vi "Read byte orders.vi"(8 "error in":errorcluster, 11 "Profibus Module configuration in":refnum<class "Profibus Module configuration.lvclass">) -> (0 "error out":errorcluster, 2 "byte orders":T1[](array[typedef]), 3 "Profibus Module configuration out":refnum<class "Profibus Module configuration.lvclass">)   [LabVIEW 2013, in "Profibus Module configuration.lvclass"]
uses:
  Profibus Module configuration.lvclass
  endianness setting.ctl
  Profibus Module configuration.lvclass/Profibus Module configuration.ctl
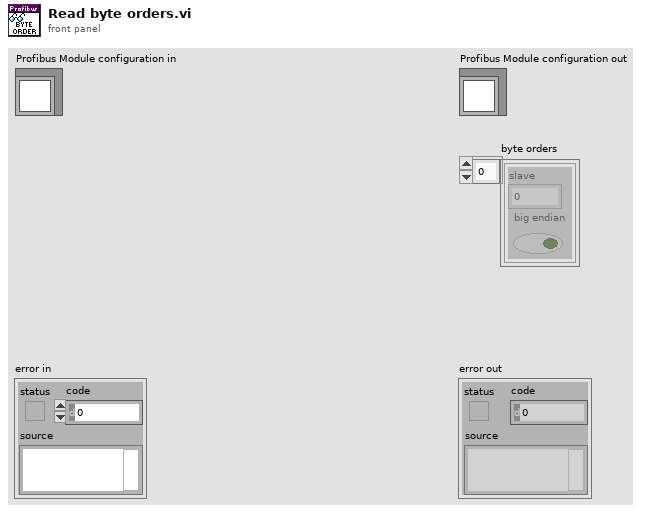
[diagram p1: front panel]
types:
  T1 = typedef "Profibus Module configuration.lvclass/endianness setting.ctl" = cluster{"slave":i8, "big endian":bool}
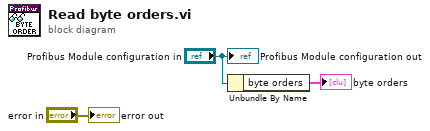
[diagram p0: block diagram]
diagram:
  n1 = Unbundle By Name("Profibus Module configuration in") -> ("byte orders"=→"byte orders":T1[])
  "error out" <- "error in"
  "Profibus Module configuration out" <- "Profibus Module configuration in"
